vi "Find PUT Center.vi"() -> ()   [LabVIEW 2019]
uses:
  Classes/Workspace/Workspace.ctl
  Classes/Workspace/Pick Up Tool Area/Pick Up Tool Fixture.lvclass
  Classes/Routine/Pick and Place/Pick and Place.lvclass
  Classes/Routine/Pick and Place/Pick and Place Type.ctl
  Classes/Routine/Pick and Place/Pick and Place.lvclass/Pick and Place.ctl
  Classes/Routine/Pick and Place/Write Pick and Place Type.vi
  Classes/Controller/Controller.lvclass
  Classes/Workspace/Fixture.lvclass
panel:
  out "Error Out":errorcluster
  in  "error in (no error)":errorcluster
  out "Workspace Out":T1
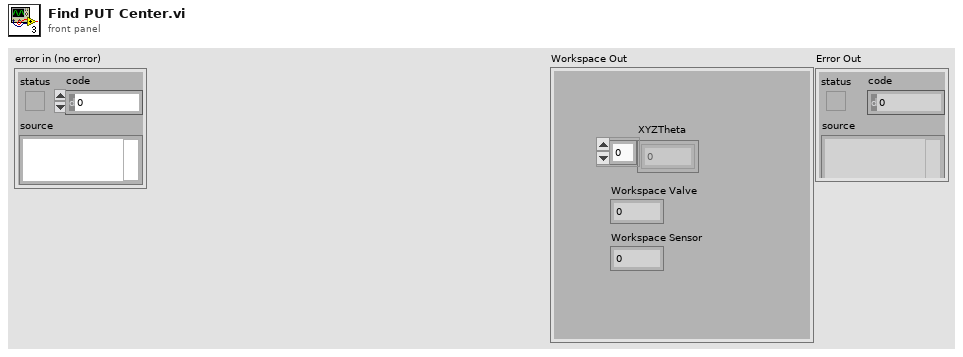
[diagram p1: front panel]
types:
  T1 = typedef "Fixture.lvclass/Workspace.ctl" = cluster{"XYZTheta":dbl[], "Workspace Valve":i32, "Workspace Sensor":i32}
  T2 = typedef "Pick and Place.lvclass/Pick and Place Type.ctl" = enum16{"Primary Pick Up", "Secondary Pick Up", "Put Down All", "Pick Up All", "Put Down Secondary"}
  T3 = typedef "Controller.lvclass/Controllers.ctl" = cluster{"I-O.lvclass":refnum<class "I-O.lvclass">, "Dispenser.lvclass":refnum<class "Dispenser.lvclass">, "Gantry":refnum<k24>}
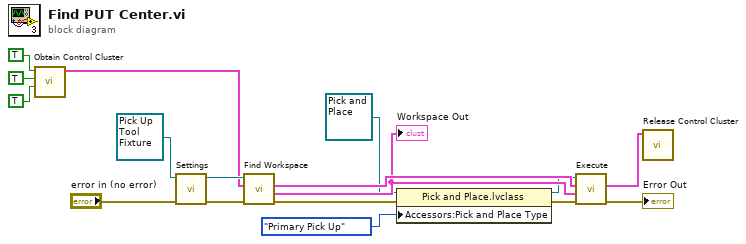
[diagram p0: block diagram]
diagram:
  n1 = call "Obtain Control Cluster.vi"("I/O"=TRUE, "Dispense"=TRUE, "Motion"=TRUE) -> ("Control Out"=w15:T3)  [unwired: 8 in]
  n2 = call-dynamic "Settings.vi"("error in (no error)"="error in (no error)", "Workspace in"=refnum<class "Pick Up Tool Fixture.lvclass"> refnum ("Pick Up Tool Fixture.lvclass")) -> ("error out"=w13:errorcluster, "Workspace out"=w16:refnum<class "Pick Up Tool Fixture.lvclass">)  [unwired: 8 in]
  n3 = call-dynamic "Find Workspace.vi"("Error In"=w13, "Control In"=w15, "Workspace In"=w16) -> ("Error Out"=w5:errorcluster, "Workspace Out"=w10:T1, "Control Out"=w11:T3)  [unwired: 5 in, 1 out]
  "Workspace Out" <- w10
  n4 = property class="Pick and Place.lvclass"(reference=refnum<class "Pick and Place.lvclass"> refnum ("Pick and Place.lvclass"), error in=w5, "Accessors:Pick and Place Type"=Pick_and_Place_Type."Primary Pick Up" ("Pick and Place Type")) -> (reference out=w7:refnum<class "Pick and Place.lvclass">, error out=w4:errorcluster)
  n5 = call-dynamic "Execute.vi"("error in (no error)"=w4, "Workspace"=w10, "Cluster"=w11, "Pick and Place in"=w7) -> ("error out"=→"Error Out":errorcluster, "Control Out"=w12:T3)  [unwired: 5 in, 1 out]
  n6 = call "Release Control Cluster.vi"("output cluster"=w12) -> ()  [unwired: 11 in]
